vi "peak comb -- interpolate - complex plane - V5.vi"(8 "chunks":T1={"start F (Hz)"=300000.0, "stop F (Hz)"=600000.0, "total number of points"=3000, "chunk size"=10, "freq step (Hz)"=0.0, "update rate (Hz)"=0.0, "adaptive parameters"={"peaks are known -- parameters"={"Def Gamma (kHz)"=0.5, "dV"=17.0, "time in Gamma (sec)"=7.0, "phi-star"=0.0, "all peaks (kHz)"=[], "delta t (sec)"=22.0, "default step (Hz)"=0.0, "all gamma (kHz)"=[564.0, 649.0, 987.0, 1133.0, 1214.0, 1585.0, 1763.0, 1823.0, 1880.0, 1899.0, 2032.0, 2138.0, 2221.0, 2270.0, 2350.0, 2456.0, 2580.0, 2634.0, 2831.0, 2960.0, 2965.0, 3131.0, 3328.0, 3469.0, 3553.0, 0.0, 3615.0, 3734.0, 0.0, 0.0, 0.0, 4236.0, 4300.0, 4331.0], "peaks OK"=FALSE, "gamma OK"=FALSE, "near omega (kHz)"=0.0, "near gamma (kHz)"=0.0, "min step (Hz)"=10000.0, "max step(Hz)"=0.01, "min gamma (kHz)"=0.01, "all time in gamma (sec)"=[], "time in gamma OK"=FALSE, "time-in-gamma mode"=enum."same for all"}, "find peak - parameters"={"wavepacket"={"R"=0.5, "wave number"=17.0, "delta k"=7.0, "radii vector"=[], "radial section"=[], "wave vector"=22.0, "wavepacket is"=TRUE}, "number of grid points"=70, "decimation threshold"=1, "Voltage range"=0.1, "target freq step"=20.0, "target spot size"=0.05, "factor"=1.0, "another factor"=1.0, "analyze last # sec"=3, "scale factor"=3}}, "total sweep time (sec)"=0.0, "chunk time (sec)"=0.0, "spot size (V)"=0.0, "uniform freq step (Hz)"=0.0, "next start freq (Hz)"=0.0} {"next start freq (Hz)" format="%#9_8f"; "uniform freq step (Hz)" format="%#_3f"; "spot size (V)" format="%#_2f"; "adaptive parameters"."find peak - parameters"."wavepacket"."delta k" format="%#_3f"; "adaptive parameters"."find peak - parameters"."wavepacket"."wave number" format="%#_3f"; "adaptive parameters"."find peak - parameters"."wavepacket"."R" format="%#_3f"; "freq step (Hz)" format="%#4_4f"; "stop F (Hz)" format="%#_3f"; "start F (Hz)" format="%#_3f"}, 11 "freq (kHz)":dbl) -> (0 "chunks OUT":T1={"start F (Hz)"=300000.0, "stop F (Hz)"=600000.0, "total number of points"=3000, "chunk size"=10, "freq step (Hz)"=0.0, "update rate (Hz)"=0.0, "adaptive parameters"={"peaks are known -- parameters"={"Def Gamma (kHz)"=0.5, "dV"=17.0, "time in Gamma (sec)"=7.0, "phi-star"=0.0, "all peaks (kHz)"=[], "delta t (sec)"=22.0, "default step (Hz)"=0.0, "all gamma (kHz)"=[564.0, 649.0, 987.0, 1133.0, 1214.0, 1585.0, 1763.0, 1823.0, 1880.0, 1899.0, 2032.0, 2138.0, 2221.0, 2270.0, 2350.0, 2456.0, 2580.0, 2634.0, 2831.0, 2960.0, 2965.0, 3131.0, 3328.0, 3469.0, 3553.0, 0.0, 3615.0, 3734.0, 0.0, 0.0, 0.0, 4236.0, 4300.0, 4331.0], "peaks OK"=FALSE, "gamma OK"=FALSE, "near omega (kHz)"=0.0, "near gamma (kHz)"=0.0, "min step (Hz)"=10000.0, "max step(Hz)"=0.01, "min gamma (kHz)"=0.01, "all time in gamma (sec)"=[], "time in gamma OK"=FALSE, "time-in-gamma mode"=enum."same for all"}, "find peak - parameters"={"wavepacket"={"R"=0.5, "wave number"=17.0, "delta k"=7.0, "radii vector"=[], "radial section"=[], "wave vector"=22.0, "wavepacket is"=TRUE}, "number of grid points"=70, "decimation threshold"=1, "Voltage range"=0.1, "target freq step"=20.0, "target spot size"=0.05, "factor"=1.0, "another factor"=1.0, "analyze last # sec"=3, "scale factor"=3}}, "total sweep time (sec)"=0.0, "chunk time (sec)"=0.0, "spot size (V)"=0.0, "uniform freq step (Hz)"=0.0, "next start freq (Hz)"=0.0} {"next start freq (Hz)" format="%#9_8f"; "uniform freq step (Hz)" format="%#_3f"; "spot size (V)" format="%#_2f"; "adaptive parameters"."find peak - parameters"."wavepacket"."delta k" format="%#_3f"; "adaptive parameters"."find peak - parameters"."wavepacket"."wave number" format="%#_3f"; "adaptive parameters"."find peak - parameters"."wavepacket"."R" format="%#_3f"; "freq step (Hz)" format="%#4_4f"; "stop F (Hz)" format="%#_3f"; "start F (Hz)" format="%#_3f"}, 1 "near omega (kHz)":dbl, 2 "near gamma (kHz)":dbl, 3 "delta-F (Hz)":dbl=-1.0)   [LabVIEW 2012]
uses:
  single sweep - frequency chunks.ctl
  single sweep - adaptive parameters.ctl
  next chunk -- parameters.ctl
  time in gamma mode control.ctl
  find peak -- parameters.ctl
  wavepacket.ctl
  Q - not nan -- real.vi
panel:
  in  "max step(Hz)":dbl=10000.0
  in  "min step (Hz)":dbl=0.01
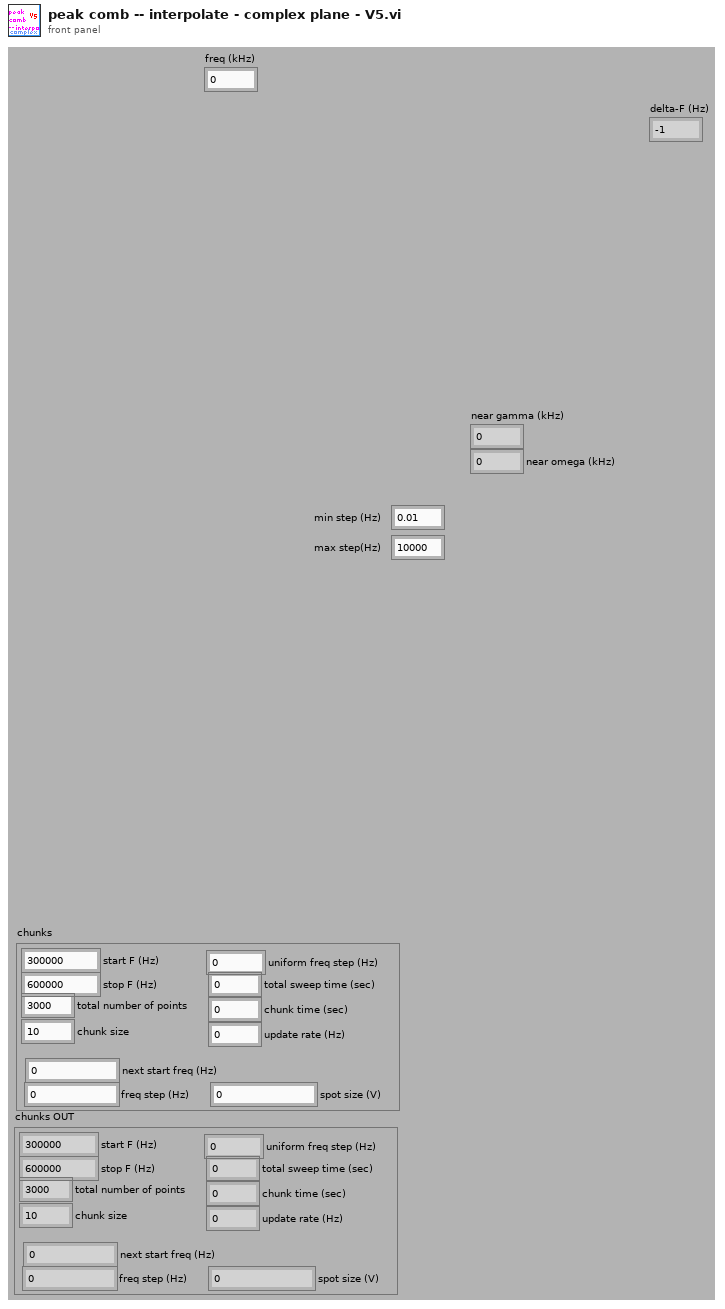
[diagram p1: front panel]
types:
  T1 = typedef "single sweep - frequency chunks.ctl" = cluster{"start F (Hz)":dbl, "stop F (Hz)":dbl, "total number of points":i32, "chunk size":i32, "freq step (Hz)":dbl, "update rate (Hz)":dbl, "adaptive parameters":T2, "total sweep time (sec)":dbl, "chunk time (sec)":dbl, "spot size (V)":dbl, "uniform freq step (Hz)":dbl, "next start freq (Hz)":dbl}
  T2 = typedef "single sweep - adaptive parameters.ctl" = cluster{"peaks are known -- parameters":T3, "find peak - parameters":T5}
  T3 = typedef "next chunk -- parameters.ctl" = cluster{"Def Gamma (kHz)":dbl, "dV":dbl, "time in Gamma (sec)":dbl, "phi-star":dbl, "all peaks (kHz)":dbl[], "delta t (sec)":dbl, "default step (Hz)":dbl, "all gamma (kHz)":dbl[], "peaks OK":bool, "gamma OK":bool, "near omega (kHz)":dbl, "near gamma (kHz)":dbl, "min step (Hz)":dbl, "max step(Hz)":dbl, "min gamma (kHz)":dbl, "all time in gamma (sec)":dbl[], "time in gamma OK":bool, "time-in-gamma mode":T4}
  T4 = typedef "time in gamma mode control.ctl" = enum16{"same for all", "each one different", "uniform scan"}
  T5 = typedef "find peak -- parameters.ctl" = cluster{"wavepacket":T6, "number of grid points":i32, "decimation threshold":i32, "Voltage range":dbl, "target freq step":dbl, "target spot size":dbl, "factor":dbl, "another factor":dbl, "analyze last # sec":i32, "scale factor":i32}
  T6 = typedef "wavepacket.ctl" = cluster{"R":dbl, "wave number":dbl, "delta k":dbl, "radii vector":dbl[], "radial section":cdb[], "wave vector":dbl, "wavepacket is":bool}
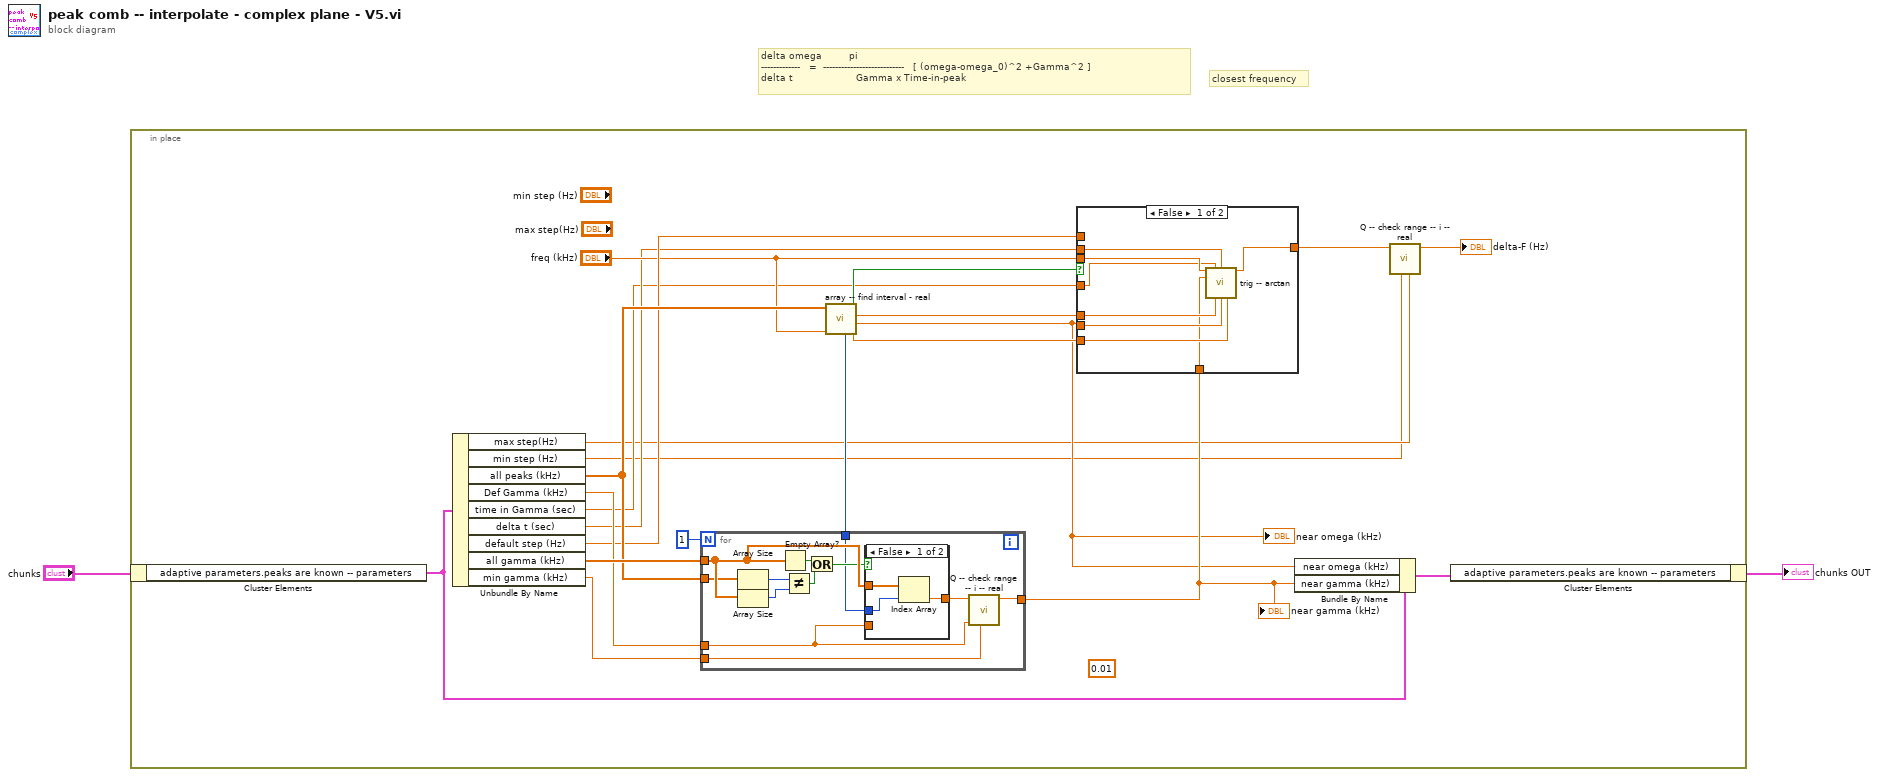
[diagram p0: block diagram]
diagram:
  # "closest frequency"
  # "delta omega         pi\n-------------   =  ---------------------------   [ (omega-omega_0)^2 +Gamma^2 ] \ndelta t                     Gamma x Time-in-peak"
  n1 = in-place {
    (unwired) 0.01 ("lower")
    n2 = in-place-cluster #1("chunks") -> ("adaptive parameters.peaks are known -- parameters"=w4:T3)
    n3 = Unbundle By Name(w4) -> ("max step(Hz)"=w8:dbl, "min step (Hz)"=w7:dbl, "all peaks (kHz)"=w20:dbl[], "Def Gamma (kHz)"=w22:dbl, "time in Gamma (sec)"=w12:dbl, "delta t (sec)"=w13:dbl, "default step (Hz)"=w18:dbl, "all gamma (kHz)"=w23:dbl[], "min gamma (kHz)"=w6:dbl)
    n4 = call "array -- find interval - real.vi"("number"="freq (kHz)", "array"=w20) -> ("omega plus (kHz)"=w16:dbl, "omega zero (kHz)"=w9:dbl, "omega minus (kHz)"=w17:dbl, "out of range?"=w19:bool, "closest element index"=w15:i32)  [unwired: 4 in, 1 out]
    "near omega (kHz)" <- w9
    n5 = for {
      N: 1 -> [_]
      tunnel: w23 -> [w34]
      tunnel: w22 -> [w28]
      tunnel: w20 -> [w27]
      tunnel: w15 -> [w26]
      tunnel: [w25] -> w10
      tunnel: w6 -> [w24]
      n6 = Array Size(array=w27) -> (size(s)=w32:i32)
      n7 = Array Size(array=w34) -> (size(s)=w33:i32)
      n8 = Empty Array?(array=w34) -> (empty?=w31:bool)
      n9 = Not Equal?(x=w32, y=w33) -> (x != y?=w30:bool)
      n10 = Or(x=w31, y=w30) -> (x .or. y?=w29:bool)
      n11 = case shown="False" w29 {
        tunnel: w26 -> [w38 _]
        tunnel: [w37 w39] -> w35
        tunnel: w34 -> [w36 _]
        tunnel: w28 -> [_ w39]
        frame False {
          n12 = Index Array(array=w36, index=w38) -> (element=w37:dbl)
        }
        frame True {
        }
      }
      n13 = call "Q -- check range -- i -- real.vi"("lower"=w24, "default"=w28, "number"=w35) -> ("number in range"=w25:dbl)  [unwired: 6 in, 2 out]
    }
    "near gamma (kHz)" <- w10
    n14 = case shown="False" w19 {
      tunnel: [w40 w48] -> w11
      tunnel: w18 -> [_ w48]
      tunnel: w17 -> [w47 _]
      tunnel: w9 -> [w46 _]
      tunnel: w16 -> [w45 _]
      tunnel: w10 -> [w44 _]
      tunnel: "freq (kHz)" -> [w43 _]
      tunnel: w13 -> [w42 _]
      tunnel: w12 -> [w41 _]
      frame False {
        n15 = call "trig -- arctan.vi"("omega (kHz)"=w43, "time in Gamma (sec)"=w41, "delta t (sec)"=w42, "gamma (kHz)"=w44, "omega minus (kHz)"=w47, "omega zero (kHz)"=w46, "omega plus (kHz)"=w45) -> ("freq step (Hz)"=w40:dbl)  [unwired: 8 in]
      }
      frame True {
      }
    }
    n16 = Bundle By Name(cluster=w4, "near omega (kHz)"=w9, "near gamma (kHz)"=w10) -> (w3:T3)
    n17 = call "Q -- check range -- i -- real.vi"("upper"=w8, "lower"=w7, "number"=w11) -> ("number in range"=→"delta-F (Hz)":dbl)  [unwired: 6 in, 2 out]
    n18 = in-place-cluster #1("adaptive parameters.peaks are known -- parameters"=w3) -> (→"chunks OUT":T1)
  }
